vi "RemoveOldBusNumber.vi"(8 "ErrorArray In":errorcluster[](array[cluster])) -> (0 "ErrorArray Out":errorcluster[](array[cluster]))   [LabVIEW 2017, in "Framework.lvlib"]
uses:
  Framework.lvlib
  <userlib>/NIST/NISTErrorLib/NISTErrorLib.lvlib
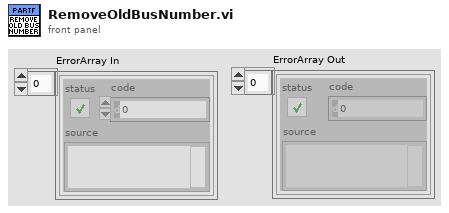
[diagram p1: front panel]
types:
  T1 = typedef "Framework.lvlib/clFrontPanelControlRefs.ctl" = cluster{"TestFilePathRef":refnum<vi>, "BusNumberRef":refnum<vi>, "NumberOfBusesRef":refnum<vi>, "EvtTypeRef":refnum<vi>, "EvtParamsRef":refnum<vi>, "EvtConfigRef":refnum<vi>, "StartTimeRef":refnum<vi>, "EndTimeRef":refnum<vi>, "PmuImpairTypeRef":refnum<vi>, "PmuImpairParamsRef":refnum<vi>, "NetImpairParamsRef":refnum<vi>, "FlagImpairTypeRef":refnum<vi>, "FlagImpairParamsRef":refnum<vi>, "NetImpairTypeRef":refnum<vi>, "OutputFileType":refnum<vi>, "PmuImpairConfigRef":refnum<vi>, "AppTypeRef":refnum<vi>, "ScriptPathRef":refnum<vi>, "ShowPanels?":refnum<vi>}
  T2 = typedef "LVStringsAndValuesArrayTypeDef_U8.ctl" = cluster{"String":string, "Value":u8}[]
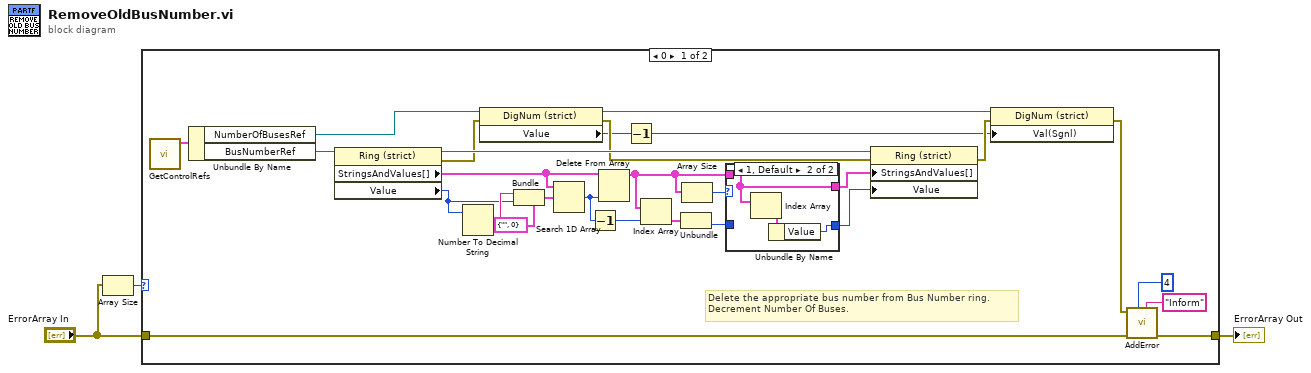
[diagram p0: block diagram]
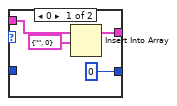
[diagram p2: hidden frame]
diagram:
  n1 = Array Size(array="ErrorArray In") -> (size(s)=w1:i32)
  n2 = case shown="0" w1 {
    tunnel: "ErrorArray In" -> [w22 w39]
    tunnel: [w21 w39] -> w2
    frame 0 {
      # "Delete the appropriate bus number from Bus Number ring.\nDecrement Number Of Buses."
      n3 = call "GetControlRefs.vi"() -> ("clControlRefs Out"=w9:T1)  [unwired: 11 in]
      n4 = Unbundle By Name(w9) -> ("NumberOfBusesRef"=w18:refnum<vi>, "BusNumberRef"=w31:refnum<vi>)
      n5 = property class="Ring (strict)"(reference=w31) -> (reference out=w27:refnum<vi>, error out=w19:errorcluster, "StringsAndValues[]"=w13:T2, "Value"=w12:u8)  [unwired: 1 in]
      n6 = Number To Decimal String(number=w12) -> (decimal integer string=w29:string)  [unwired: 1 in]
      n7 = property class="DigNum (strict)"(reference=w18, error in=w19) -> (reference out=w16:refnum<vi>, error out=w20:errorcluster, "Value"=w17:u8)
      n8 = Bundle(cluster=cluster{"String":string, "Value":u8} {"String"="", "Value"=0} ("element"), "String"=w29, "Value"=w12) -> (w28:cluster{"String":string, "Value":u8})
      n9 = Search 1D Array(1D array=w13, element=w28) -> (index of element=w14:i32)  [unwired: 1 in]
      n10 = Decrement(x=w14) -> (x-1=w11:i32)
      n11 = Delete From Array(array=w13, index=w14) -> (array with subset deleted=w7:T2)  [unwired: 1 in, 1 out]
      n12 = Decrement(x=w17) -> (x-1=w15:u8)
      n13 = Index Array(array=w7, index=w11) -> (element=w10:cluster{"String":string, "Value":u8})
      n14 = Unbundle(w10) -> ("Value"=w5:u8)  [unwired: 1 out]
      n15 = Array Size(array=w7) -> (size(s)=w8:i32)
      n16 = case shown="1, Default" w8 {
        tunnel: w7 -> [w35 w38]
        tunnel: [w33 w38] -> w6
        tunnel: w5 -> [_ _]
        tunnel: [u8 0 ("Value") w36] -> w4
        frame 0 {
          n17 = Insert Into Array(array=w35, new element=cluster{"String":string, "Value":u8} {"String"="", "Value"=0} ("new element/subarray")) -> (w33:T2)  [unwired: 1 in]
        }
        frame 1, Default {
          n18 = Index Array(array=w38) -> (element=w37:cluster{"String":string, "Value":u8})  [unwired: 1 in]
          n19 = Unbundle By Name(w37) -> ("Value"=w36:u8)
        }
      }
      n20 = property class="Ring (strict)"(reference=w27, error in=w20, "StringsAndValues[]"=w6, "Value"=w4) -> (error out=w26:errorcluster)  [unwired: 1 out]
      n21 = property class="DigNum (strict)"(reference=w16, error in=w26, "Val(Sgnl)"=w15) -> (error out=w23:errorcluster)  [unwired: 1 out]
      n22 = call <userlib>:"AddError.vi"("Severity"="Inform" ("String"), "Priority"=u8 4, "ErrorArray"=w22, "error in (no error)"=w23) -> ("ErrorArray"=w21:errorcluster[])  [unwired: 6 in, 1 out]
    }
    frame 1, Default {
    }
  }
  "ErrorArray Out" <- w2
